vi "Flatten JSON 1.0.vi"(8 "error in (no error)":errorcluster, 11 "group configurations":T1(array[cluster])) -> (0 "error out":errorcluster, 3 "JSON string":string)   [LabVIEW 2017, in "DSF Core.lvlib" / "Core Groups Configuration.lvclass"]
uses:
  Core Groups Configuration.lvclass
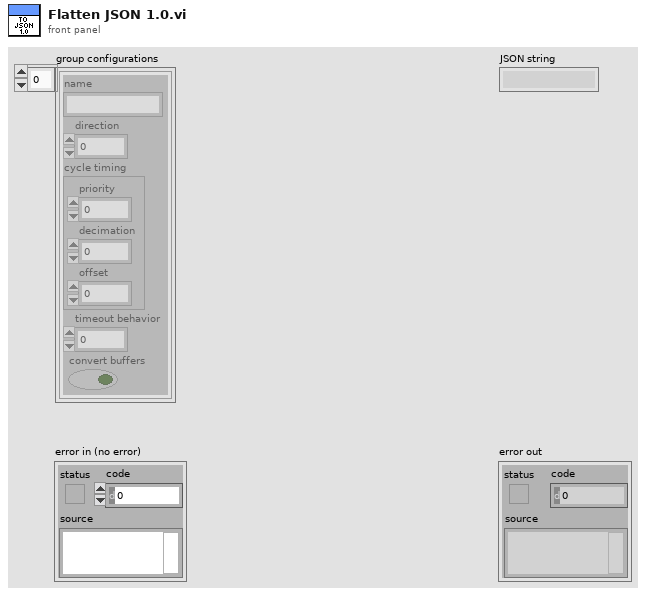
[diagram p1: front panel]
types:
  T1 = cluster{"name":string, "direction":u8, "cycle timing":cluster{"priority":u64, "decimation":u64, "offset":u64}, "timeout behavior":u8, "convert buffers":bool}[]
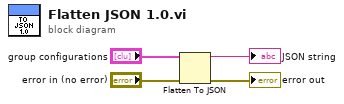
[diagram p0: block diagram]
diagram:
  n1 = Flatten To JSON(anything="group configurations", error in (no error)="error in (no error)") -> (JSON string=→"JSON string":string, 11:→"error out":errorcluster)  [unwired: 1 in]
